vi "HEWH Disable Flow Adjust.vi"(6 "State in":T1, 8 "error in (no error)":errorcluster, 10 "GPM Target":T2 format="%.2f", 11 "Elapsed Time (sec) in":dbl) -> (0 "error out":errorcluster, 3 "Adjust Flow?":bool)   [LabVIEW 2020]
uses:
  Utility/Custom Pallet Controls/Custom Pallet DBL.ctl
  Type Definitions/HEWH Purge Draw.ctl
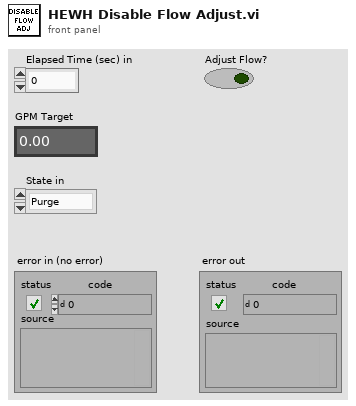
[diagram p1: front panel]
types:
  T1 = typedef "HEWH Purge Draw.ctl" = enum16{"Purge", "Draw"}
  T2 = typedef "Custom Pallet DBL.ctl" = dbl
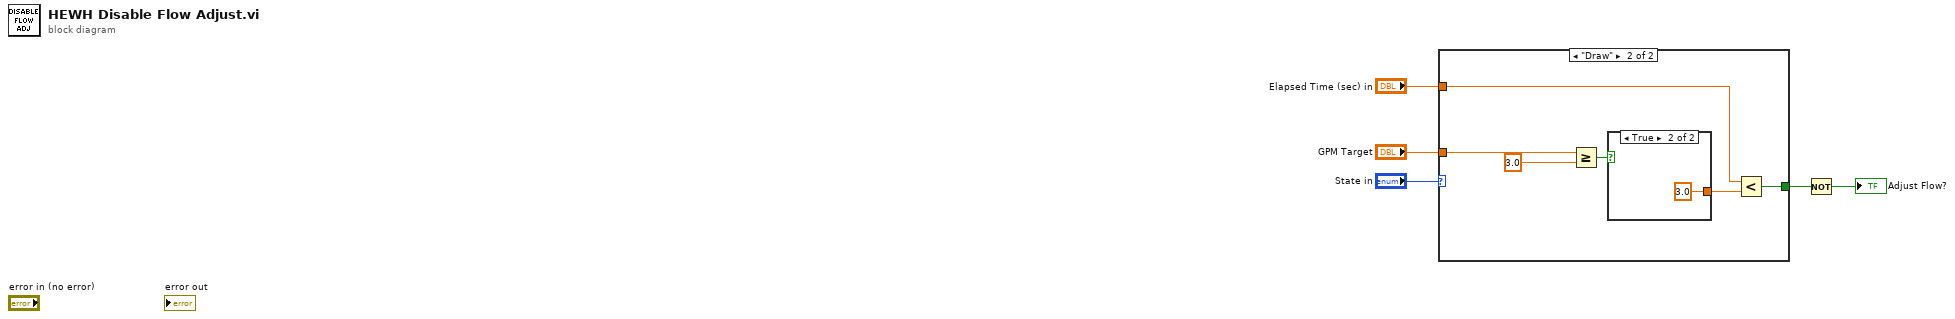
[diagram p0: block diagram]
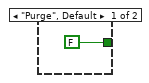
[diagram p2: hidden frame]
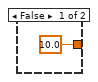
[diagram p3: hidden frame]
diagram:
  n1 = case shown="\"Draw\"" "State in" {
    tunnel: [FALSE w8] -> w2
    tunnel: "Elapsed Time (sec) in" -> [_ w10]
    tunnel: "GPM Target" -> [_ w7]
    frame "Purge", Default {
    }
    frame "Draw" {
      n2 = Greater Or Equal?(x=w7, y=3.0) -> (x >= y?=w11:bool)
      n3 = case shown="True" w11 {
        tunnel: [10.0 ("y") 3.0 ("y")] -> w12
        frame False {
        }
        frame True {
        }
      }
      n4 = Less?(x=w10, y=w12) -> (x < y?=w8:bool)
    }
  }
  n5 = Not(x=w2) -> (.not. x?=→"Adjust Flow?":bool)
